vi "Mutate 1.3.4.vi"(8 "error in (no error)":errorcluster, 11 "Device Ref in":T1 format="%.0x") -> (0 "error out":errorcluster, 2 "Skip Version Bump?":bool, 3 "Device Ref out":T1 format="%.0x")   [LabVIEW 2015, in "Engine Simulation Toolkit System Explorer.lvlib"]
uses:
  Engine Simulation Toolkit System Explorer.lvlib
  <vilib>/NI Veristand/Custom Device API/Custom Device Item Ref.ctl
  Shared/Constants and GUIDs.vi
  Shared/Properties.vi
  <vilib>/NI Veristand/Custom Device API/Get Item Property (Boolean).vi
  <vilib>/NI Veristand/Custom Device API/Get Item Property (String).vi
  <vilib>/NI Veristand/Custom Device API/Set Item Property (String Array).vi
  <vilib>/NI Veristand/Custom Device API/Get Item Property (Dependent File).vi
  <vilib>/NI Veristand/Custom Device API/Set Item Property (String).vi
  <vilib>/NI Veristand/Custom Device Tools/Custom Device Utility Library/NI VeriStand - Search for Item by GUID.vi
  Shared/Engine Simulation Toolkit Shared.lvlib
  <vilib>/NI VeriStand/Custom Device API/Custom Device API.lvlib
  <vilib>/NI VeriStand/Custom Device Tools/Custom Device Utility Library/Custom Device Utility Library.lvlib
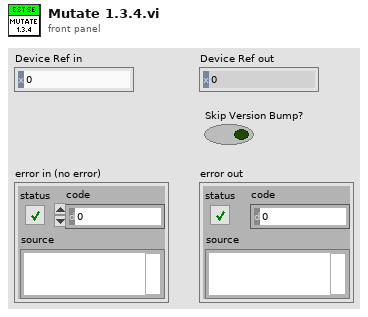
[diagram p1: front panel]
types:
  T1 = typedef "Custom Device API.lvlib/Custom Device Item Ref.ctl" = u64
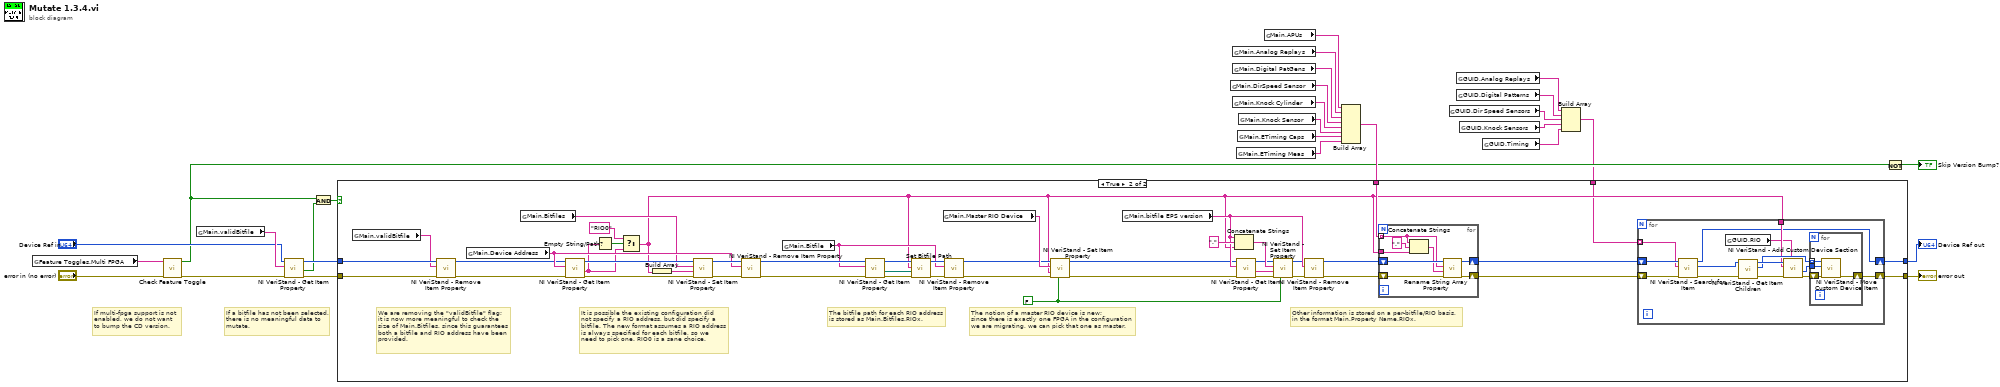
[diagram p0: block diagram]
diagram:
  # "If multi-fpga support is not\nenabled, we do not want\nto bump the CD version."
  # "If a bitfile has not been selected,\nthere is no meaningful data to\nmutate."
  n1 = global read "Constants and GUIDs.vi" "Feature Toggles.Multi FPGA"() -> (w28:string)
  n2 = call "Check Feature Toggle.vi"("error in (no error)"="error in (no error)", "feature name"=w28) -> ("error out"=w13:errorcluster, "feature enabled"=w7:bool)  [unwired: 8 in]
  n3 = global read "Properties.vi" "Main.validBitfile"() -> (w14:string)
  n4 = call-poly <vilib>:"NI VeriStand - Get Item Property.vi"("error in (no error)"=w13, "Property Name"=w14, "Item Ref in"="Device Ref in") -> ("error out"=w12:errorcluster, "Value"=w8:bool, "Item Ref out"=w11:T1)  [unwired: 5 in, 1 out]
  n5 = And(x=w7, y=w8) -> (x .and. y?=w9:bool)
  n6 = global read "Properties.vi" "Main.DirSpeed Sensor"() -> (w19:string)
  n7 = global read "Properties.vi" "Main.Analog Replays"() -> (w17:string)
  n8 = global read "Properties.vi" "Main.Digital PatGens"() -> (w18:string)
  n9 = global read "Properties.vi" "Main.Knock Cylinder"() -> (w20:string)
  n10 = global read "Properties.vi" "Main.ETiming Meas"() -> (w22:string)
  n11 = global read "Properties.vi" "Main.ETiming Caps"() -> (w21:string)
  n12 = global read "Properties.vi" "Main.Knock Sensor"() -> (w23:string)
  n13 = global read "Properties.vi" "Main.APUs"() -> (w16:string)
  n14 = Build Array(w16, w17, w18, w19, w20, w23, w21, w22) -> (w15:string[])
  n15 = global read "Constants and GUIDs.vi" "GUID.Dir Speed Sensors"() -> (w4:string)
  n16 = global read "Constants and GUIDs.vi" "GUID.Analog Replays"() -> (w2:string)
  n17 = global read "Constants and GUIDs.vi" "GUID.Digital Patterns"() -> (w3:string)
  n18 = global read "Constants and GUIDs.vi" "GUID.Knock Sensors"() -> (w5:string)
  n19 = global read "Constants and GUIDs.vi" "GUID.Timing"() -> (w6:string)
  n20 = Build Array(w2, w3, w4, w5, w6) -> (w1:string[])
  n21 = case shown="True" w9 {
    tunnel: w12 -> [w29 w37]
    tunnel: w11 -> [w30 w41]
    tunnel: [w30 w32] -> w25
    tunnel: [w29 w33] -> w24
    tunnel: w15 -> [_ w53]
    tunnel: w1 -> [_ w31]
    frame False {
    }
    frame True {
      w42 = FALSE ("Binary String (T)")
      # "We are removing the \"validBitfile\" flag;\nit is now more meaningful to check the\nsize of Main.Bitfiles, since this guarantees\nboth a bitfile and RIO address have been\nprovided."
      # "Other information is stored on a per-bitfile/RIO basis,\nin the format Main.Property Name.RIOx."
      # "The notion of a master RIO device is new;\nsince there is exactly one FPGA in the configuration\nwe are migrating, we can pick that one as master."
      # "The bitfile path for each RIO address\nis stored as Main.Bitfiles.RIOx."
      # "It is possible the existing configuration did\nnot specify a RIO address, but did specify a\nbitfile. The new format assumes a RIO address\nis always specified for each bitfile, so we\nneed to pick one. RIO0 is a sane choice."
      n22 = global read "Properties.vi" "Main.validBitfile"() -> (w40:string)
      n23 = call <vilib>:"NI VeriStand - Remove Item Property.vi"("error in (no error)"=w37, "Property Name"=w40, "Item Ref in"=w41) -> ("error out"=w38:errorcluster, "Item Ref out"=w39:T1)  [unwired: 6 in, 1 out]
      n24 = global read "Properties.vi" "Main.Device Address"() -> (w68:string)
      n25 = global read "Properties.vi" "Main.Bitfiles"() -> (w54:string)
      n26 = call-poly <vilib>:"NI VeriStand - Get Item Property.vi"("error in (no error)"=w38, "Property Name"=w68, "Item Ref in"=w39) -> ("error out"=w74:errorcluster, "Value"=w51:string, "Item Ref out"=w75:T1)  [unwired: 5 in, 1 out]
      n27 = Empty String/Path?(string/path=w51) -> (empty?=w52:bool)
      n28 = Select(t="RIO0", s=w52, f=w51) -> (s? t:f=w36:string)
      n29 = Build Array(w36) -> (w76:string[])
      n30 = call-poly <vilib>:"NI VeriStand - Set Item Property.vi"("error in (no error)"=w74, "Value"=w76, "Property Name"=w54, "Item Ref in"=w75) -> ("error out"=w69:errorcluster, "Item Ref out"=w70:T1)  [unwired: 5 in, 1 out]
      n31 = call <vilib>:"NI VeriStand - Remove Item Property.vi"("error in (no error)"=w69, "Property Name"=w68, "Item Ref in"=w70) -> ("error out"=w66:errorcluster, "Item Ref out"=w67:T1)  [unwired: 6 in, 1 out]
      n32 = global read "Properties.vi" "Main.Bitfile"() -> (w63:string)
      n33 = call-poly <vilib>:"NI VeriStand - Get Item Property.vi"("error in (no error)"=w66, "Property Name"=w63, "Item Ref in"=w67) -> ("error out"=w73:errorcluster, "Path"=w72:path, "Item Ref out"=w71:T1)  [unwired: 4 in, 2 out]
      n34 = call "Set Bitfile Path.vi"("error in (no error)"=w73, "Bitfile Path in"=w72, "RIO Device Address in"=w36, "Item Ref in"=w71) -> ("error out"=w65:errorcluster, "Item Ref out"=w64:T1)  [unwired: 6 in]
      n35 = global read "Properties.vi" "Main.Master RIO Device"() -> (w47:string)
      n36 = call <vilib>:"NI VeriStand - Remove Item Property.vi"("error in (no error)"=w65, "Property Name"=w63, "Item Ref in"=w64) -> ("error out"=w45:errorcluster, "Item Ref out"=w44:T1)  [unwired: 6 in, 1 out]
      n37 = call-poly <vilib>:"NI VeriStand - Set Item Property.vi"("Binary String (T)"=w42, "error in (no error)"=w45, "Value"=w36, "Property Name"=w47, "Item Ref in"=w44) -> ("error out"=w46:errorcluster, "Item Ref out"=w43:T1)  [unwired: 4 in, 1 out]
      n38 = global read "Properties.vi" "Main.bitfile EPS version"() -> (w58:string)
      n39 = Concatenate Strings(w58, "." ("string"), w36) -> (w59:string)
      n40 = call-poly <vilib>:"NI VeriStand - Get Item Property.vi"("error in (no error)"=w46, "Property Name"=w58, "Item Ref in"=w43) -> ("error out"=w61:errorcluster, "Value"=w60:string, "Item Ref out"=w57:T1)  [unwired: 5 in, 1 out]
      n41 = call-poly <vilib>:"NI VeriStand - Set Item Property.vi"("Binary String (T)"=w42, "error in (no error)"=w61, "Value"=w60, "Property Name"=w59, "Item Ref in"=w57) -> ("error out"=w55:errorcluster, "Item Ref out"=w56:T1)  [unwired: 4 in, 1 out]
      n42 = call <vilib>:"NI VeriStand - Remove Item Property.vi"("error in (no error)"=w55, "Property Name"=w58, "Item Ref in"=w56) -> ("error out"=w49:errorcluster, "Item Ref out"=w48:T1)  [unwired: 6 in, 1 out]
      n43 = for {
        tunnel: w36 -> [w101]
        tunnel: w53 -> [w98] mode=indexing
        shift-right: [w96] -> w34
        shift-left: w49 -> [w100]
        shift-right: [w95] -> w35
        shift-left: w48 -> [w99]
        n44 = Concatenate Strings(w98, "." ("string"), w101) -> (w97:string)
        n45 = call "Rename String Array Property.vi"("error in (no error)"=w100, "New Name"=w97, "Old Name"=w98, "Item Ref in"=w99) -> ("error out"=w96:errorcluster, "Item Ref out"=w95:T1)  [unwired: 6 in]
      }
      n46 = for {
        tunnel: w36 -> [w83]
        shift-right: [w79] -> w33
        shift-left: w34 -> [w80]
        shift-right: [w78] -> w32
        shift-left: w35 -> [w81]
        tunnel: w31 -> [w77] mode=indexing
        n47 = call-poly <vilib>:"NI VeriStand - Search for Item.vi"("error in"=w80, "Item GUID"=w77, "Section Ref in"=w81) -> ("error out"=w87:errorcluster, "Item Ref"=w90:T1, "Section Ref out"=w78:T1)  [unwired: 5 in, 1 out]
        n48 = global read "Constants and GUIDs.vi" "GUID.RIO"() -> (w82:string)
        n49 = call <vilib>:"NI VeriStand - Get Item Children.vi"("error in (no error)"=w87, "Item Ref in"=w90) -> ("error out"=w89:errorcluster, "Child Refs"=w84:T1[], "Item Ref out"=w88:T1)  [unwired: 6 in, 1 out]
        n50 = call <vilib>:"NI VeriStand - Add Custom Device Section.vi"("GUID (Default Section)"=w82, "error in (no error)"=w89, "Section Name"=w83, "Parent Ref in"=w88) -> ("error out"=w85:errorcluster, "Section Ptr"=w86:T1)  [unwired: 4 in, 2 out]
        n51 = for {
          tunnel: w86 -> [w94]
          tunnel: w84 -> [w92] mode=indexing
          shift-right: [w91] -> w79
          shift-left: w85 -> [w93]
          n52 = call <vilib>:"NI VeriStand - Move Custom Device Item.vi"("error in (no error)"=w93, "New Parent Ref in"=w94, "Item Ref in"=w92) -> ("error out"=w91:errorcluster)  [unwired: 6 in, 2 out]
        }
      }
    }
  }
  "Device Ref out" <- w25
  "error out" <- w24
  n53 = Not(x=w7) -> (.not. x?=→"Skip Version Bump?":bool)
